vi "DiffDriveSim_Write_Sensors.vi"(6 "Restart":bool, 8 "Right Encoder":T2, 9 "Left Encoder":T2, 10 "Diff Drive Train Sim":T11 {"m_Motor"."Jr_KgM2" format="%13.5p"; "m_Motor"."L_H" format="%13.5p"; "m_Motor"."Kt_NMPerAmp" format="%13.5p"; "m_Motor"."KvINV_RadPerSecPerVolt" format="%13.5p"; "m_Motor"."R_Ohms" format="%13.5p"; "m_Motor"."FreeSpeed_RadPerSec" format="%13.5p"; "m_Motor"."FreeCurrent_Amps" format="%13.5p"; "m_Motor"."StallCurrent_Amps" format="%13.5p"; "m_Motor"."StallTorque_NM" format="%13.5p"; "m_Motor"."nominalVoltage_Volts" format="%13.5p"}, 11 "Counts/Feet":dbl) -> (0 "Right Encoder":T1, 1 "Right Encoder":T9, 2 "Left Encoder":T1, 3 "Left Encoder":T9, 4 "Robot Pose":T6 {"ROTATION"."SIN" format="%13.4f"; "ROTATION"."COS" format="%13.4f"; "ROTATION"."VALUE" format="%13.4f"; "TRANSLATION"."Y" format="%14.3f"; "TRANSLATION"."X" format="%14.3f"}, 5 "Gyro Deg":dbl, 7 "Gyro":T4)   [LabVIEW 2019]
uses:
  <vilib>/Rock Robotics/WPI/ThirdParty/JAS_Junk/TrajLib/TypeDef/DIFF_DRIVE_TRAIN_SIM.ctl
  <vilib>/Rock Robotics/WPI/ThirdParty/JAS_Junk/TrajLib/TypeDef/LINEAR_SYSTEM.ctl
  <vilib>/Analysis/Matrix/Datatypes/RealMatrix.ctl
  <vilib>/Rock Robotics/WPI/ThirdParty/JAS_Junk/TrajLib/TypeDef/DCMOTOR.CTL
  <vilib>/Rock Robotics/WPI/Simulation/Protocol/Devices/Encoder/Encoder proto.ctl
  <vilib>/Rock Robotics/WPI/Simulation/Protocol/Devices/Encoder/Encoder data protoo.ctl
  <vilib>/Rock Robotics/WPI/ThirdParty/JAS_Junk/TrajLib/TypeDef/POSE2D.ctl
  <vilib>/Rock Robotics/WPI/ThirdParty/JAS_Junk/TrajLib/TypeDef/TRANSLATION2D.ctl
  <vilib>/Rock Robotics/WPI/ThirdParty/JAS_Junk/TrajLib/TypeDef/ROTATION2D.ctl
  <vilib>/Rock Robotics/WPI/Simulation/Protocol/Devices/Gyro/Gyro proto.ctl
  <vilib>/Rock Robotics/WPI/Simulation/Protocol/Devices/Gyro/Gyro Data proto.ctl
  DiffDriveSim_EncoderDIOType.ctl
  <vilib>/Rock Robotics/SystemInterfaces/DIO/FPGA_DIOChannel.ctl
  DiffDriveSim_EncoderValues.ctl
  <vilib>/Rock Robotics/WPI/Simulation/Protocol/Devices/Gyro/Gyro Update Ops.ctl
  <vilib>/Rock Robotics/WPI/Simulation/Protocol/Devices/Encoder/Encoder Values.ctl
  <vilib>/Rock Robotics/WPI/Simulation/Protocol/Devices/Encoder/Encoder Update Ops.ctl
  DiffDriveSim_GetAllEncoderInx.vi
  <vilib>/Rock Robotics/SystemInterfaces/FPGA_NIFPGAInterfaceFPGAResourceConstant.vi
  <vilib>/Rock Robotics/SystemInterfaces/Encoder/FPGA_EncoderIdx.ctl
  <vilib>/Rock Robotics/WPI/ThirdParty/JAS_Junk/TrajLib/Trajectory_Library.lvlib
  <vilib>/Analysis/Matrix/NI_Matrix.lvlib
panel:
  out "Right Enc Found":bool
  out "Left Enc Found":bool
  # "<States, 1>"
  # "<Outputs, 1>"
  # "<Inputs, 1>"
  # "<Outputs, 1>"
  # "<States,States>"
  # "<States,Inputs>"
  # "<Outputs,States>"
  # "<Outputs,Inputs>"
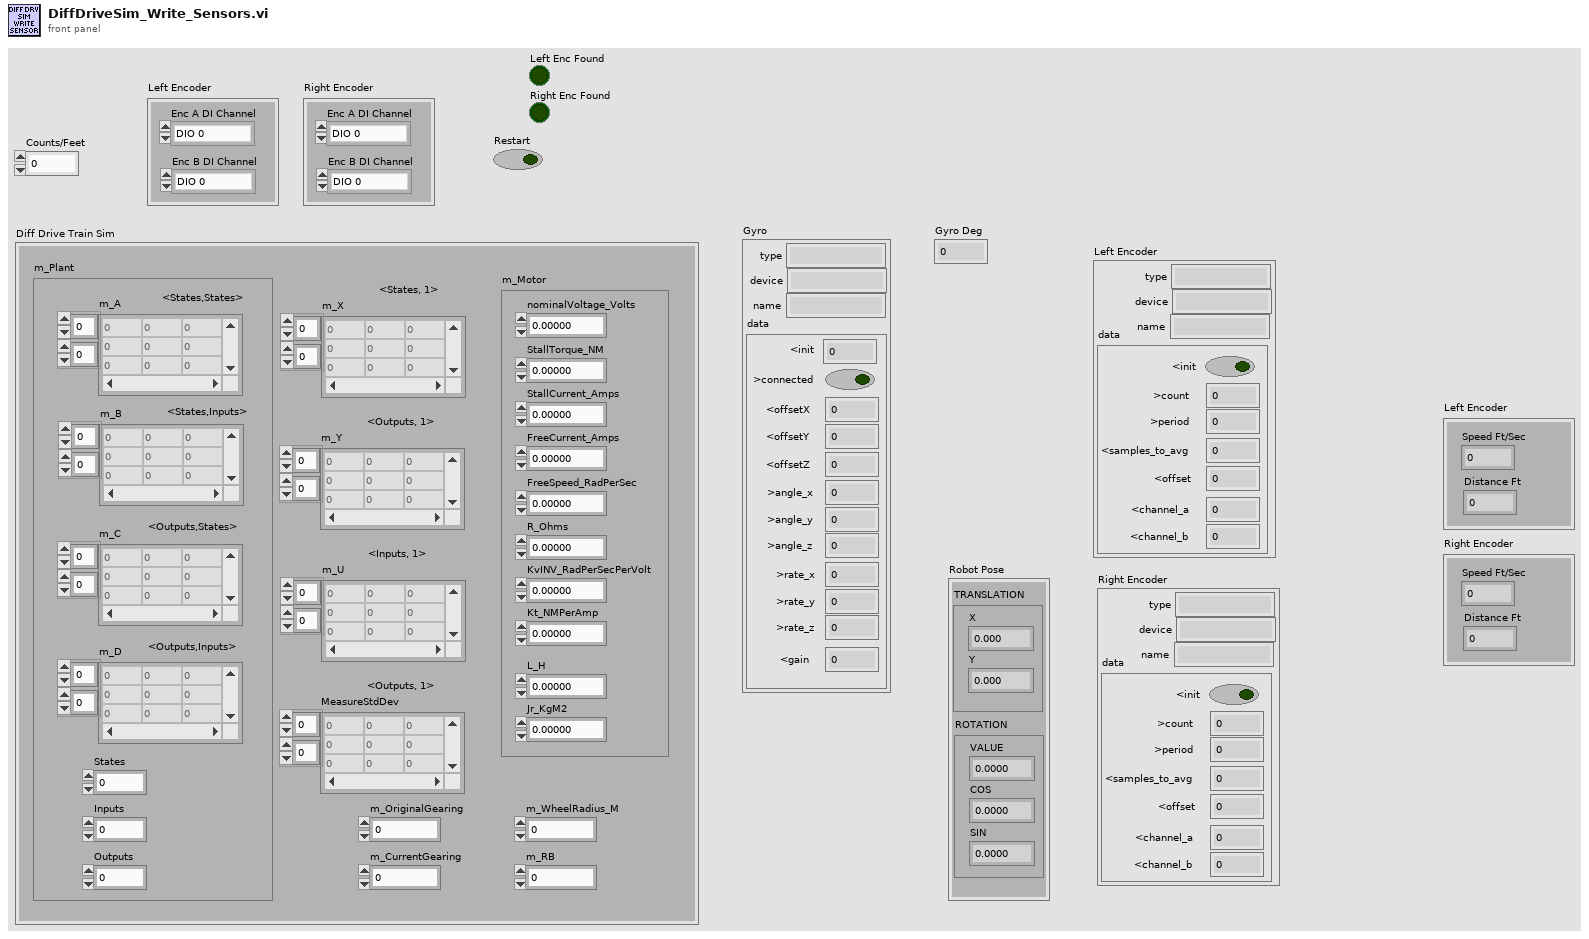
[diagram p1: front panel]
types:
  T1 = typedef "DiffDriveSim_EncoderValues.ctl" = cluster{"Speed Ft/Sec":dbl, "Distance Ft":dbl}
  T2 = typedef "DiffDriveSim_EncoderDIOType.ctl" = cluster{"Enc A DI Channel":T3, "Enc B DI Channel":T3}
  T3 = typedef "FPGA_DIOChannel.ctl" = enum8{"DIO 0", "DIO 1", "DIO 2", "DIO 3", "DIO 4", "DIO 5", "DIO 6", "DIO 7", "DIO 8", "DIO 9", "DIO MXP 0", "DIO MXP 1", "DIO MXP 2", "DIO MXP 3", "DIO MXP 4", "DIO MXP 5", "DIO MXP 6", "DIO MXP 7", "DIO MXP 8", "DIO MXP 9", "DIO MXP 10", "DIO MXP 11", "DIO MXP 12", "DIO MXP 13", "DIO MXP 14", "DIO MXP 15", "SPI Port CS1", "SPI Port CS2", "SPI Port CS3", "SPI Port MISO", "SPI Port MOSI", "Invalid"}
  T4 = typedef "Gyro proto.ctl" = cluster{"type":string, "device":string, "name":string, "data":T5}
  T5 = typedef "Gyro Data proto.ctl" = cluster{"<init":i32, ">connected":bool, "<offsetX":dbl, "<offsetY":dbl, "<offsetZ":dbl, ">angle_x":dbl, ">angle_y":dbl, ">angle_z":dbl, ">rate_x":dbl, ">rate_y":dbl, ">rate_z":dbl, "<gain":dbl}
  T6 = typedef "Trajectory_Library.lvlib/POSE2D.ctl" = cluster{"TRANSLATION":T7, "ROTATION":T8}
  T7 = typedef "Trajectory_Library.lvlib/TRANSLATION2D.ctl" = cluster{"X":dbl, "Y":dbl}
  T8 = typedef "Trajectory_Library.lvlib/ROTATION2D.ctl" = cluster{"VALUE":dbl, "COS":dbl, "SIN":dbl}
  T9 = typedef "Encoder proto.ctl" = cluster{"type":string, "device":string, "name":string, "data":T10}
  T10 = typedef "Encoder data protoo.ctl" = cluster{"<init":bool, ">count":dbl, ">period":dbl, "<samples_to_avg":i32, "<offset":dbl, "<channel_a":i32, "<channel_b":i32}
  T11 = typedef "Trajectory_Library.lvlib/DIFF_DRIVE_TRAIN_SIM.ctl" = cluster{"m_Plant":T12, "m_X":T13, "m_Y":T13, "m_U":T13, "MeasureStdDev":T13, "m_Motor":T14, "m_OriginalGearing":dbl, "m_CurrentGearing":dbl, "m_WheelRadius_M":dbl, "m_RB":dbl}
  T12 = typedef "Trajectory_Library.lvlib/LINEAR_SYSTEM.ctl" = cluster{"m_A":T13, "m_B":T13, "m_C":T13, "m_D":T13, "States":i32, "Inputs":i32, "Outputs":i32}
  T13 = typedef "NI_Matrix.lvlib/RealMatrix.ctl" = dbl[][]
  T14 = typedef "Trajectory_Library.lvlib/DCMOTOR.CTL" = cluster{"nominalVoltage_Volts":dbl, "StallTorque_NM":dbl, "StallCurrent_Amps":dbl, "FreeCurrent_Amps":dbl, "FreeSpeed_RadPerSec":dbl, "R_Ohms":dbl, "KvINV_RadPerSecPerVolt":dbl, "Kt_NMPerAmp":dbl, "L_H":dbl, "Jr_KgM2":dbl}
  T15 = typedef "Gyro Update Ops.ctl" = enum16{"get", "delete", "JSON update", "set  name", "transmit initial", "reset", "set init", "set offsetX", "set offsetY", "set offsetZ", "set gain", "set angle X", "set angle Y", "set angle Z", "set rate X", "set rate Y", "set rate Z"}
  T16 = typedef "Encoder Update Ops.ctl" = enum16{"set init", "set count", "set period", "set reset", "set samples_to_avg", "get", "delete", "JSON update", "set name", "transmit initial", "reset", "set channel_a", "set channel_b", "set values"}
  T17 = typedef "FPGA_EncoderIdx.ctl" = enum8{"Enc 0", "Enc 1", "Enc 2", "Enc 3", "Enc 4", "Enc 5", "Enc 6", "Enc 7", "Invalid"}
  T18 = typedef "Encoder Values.ctl" = cluster{"Count":dbl, "Period":dbl}
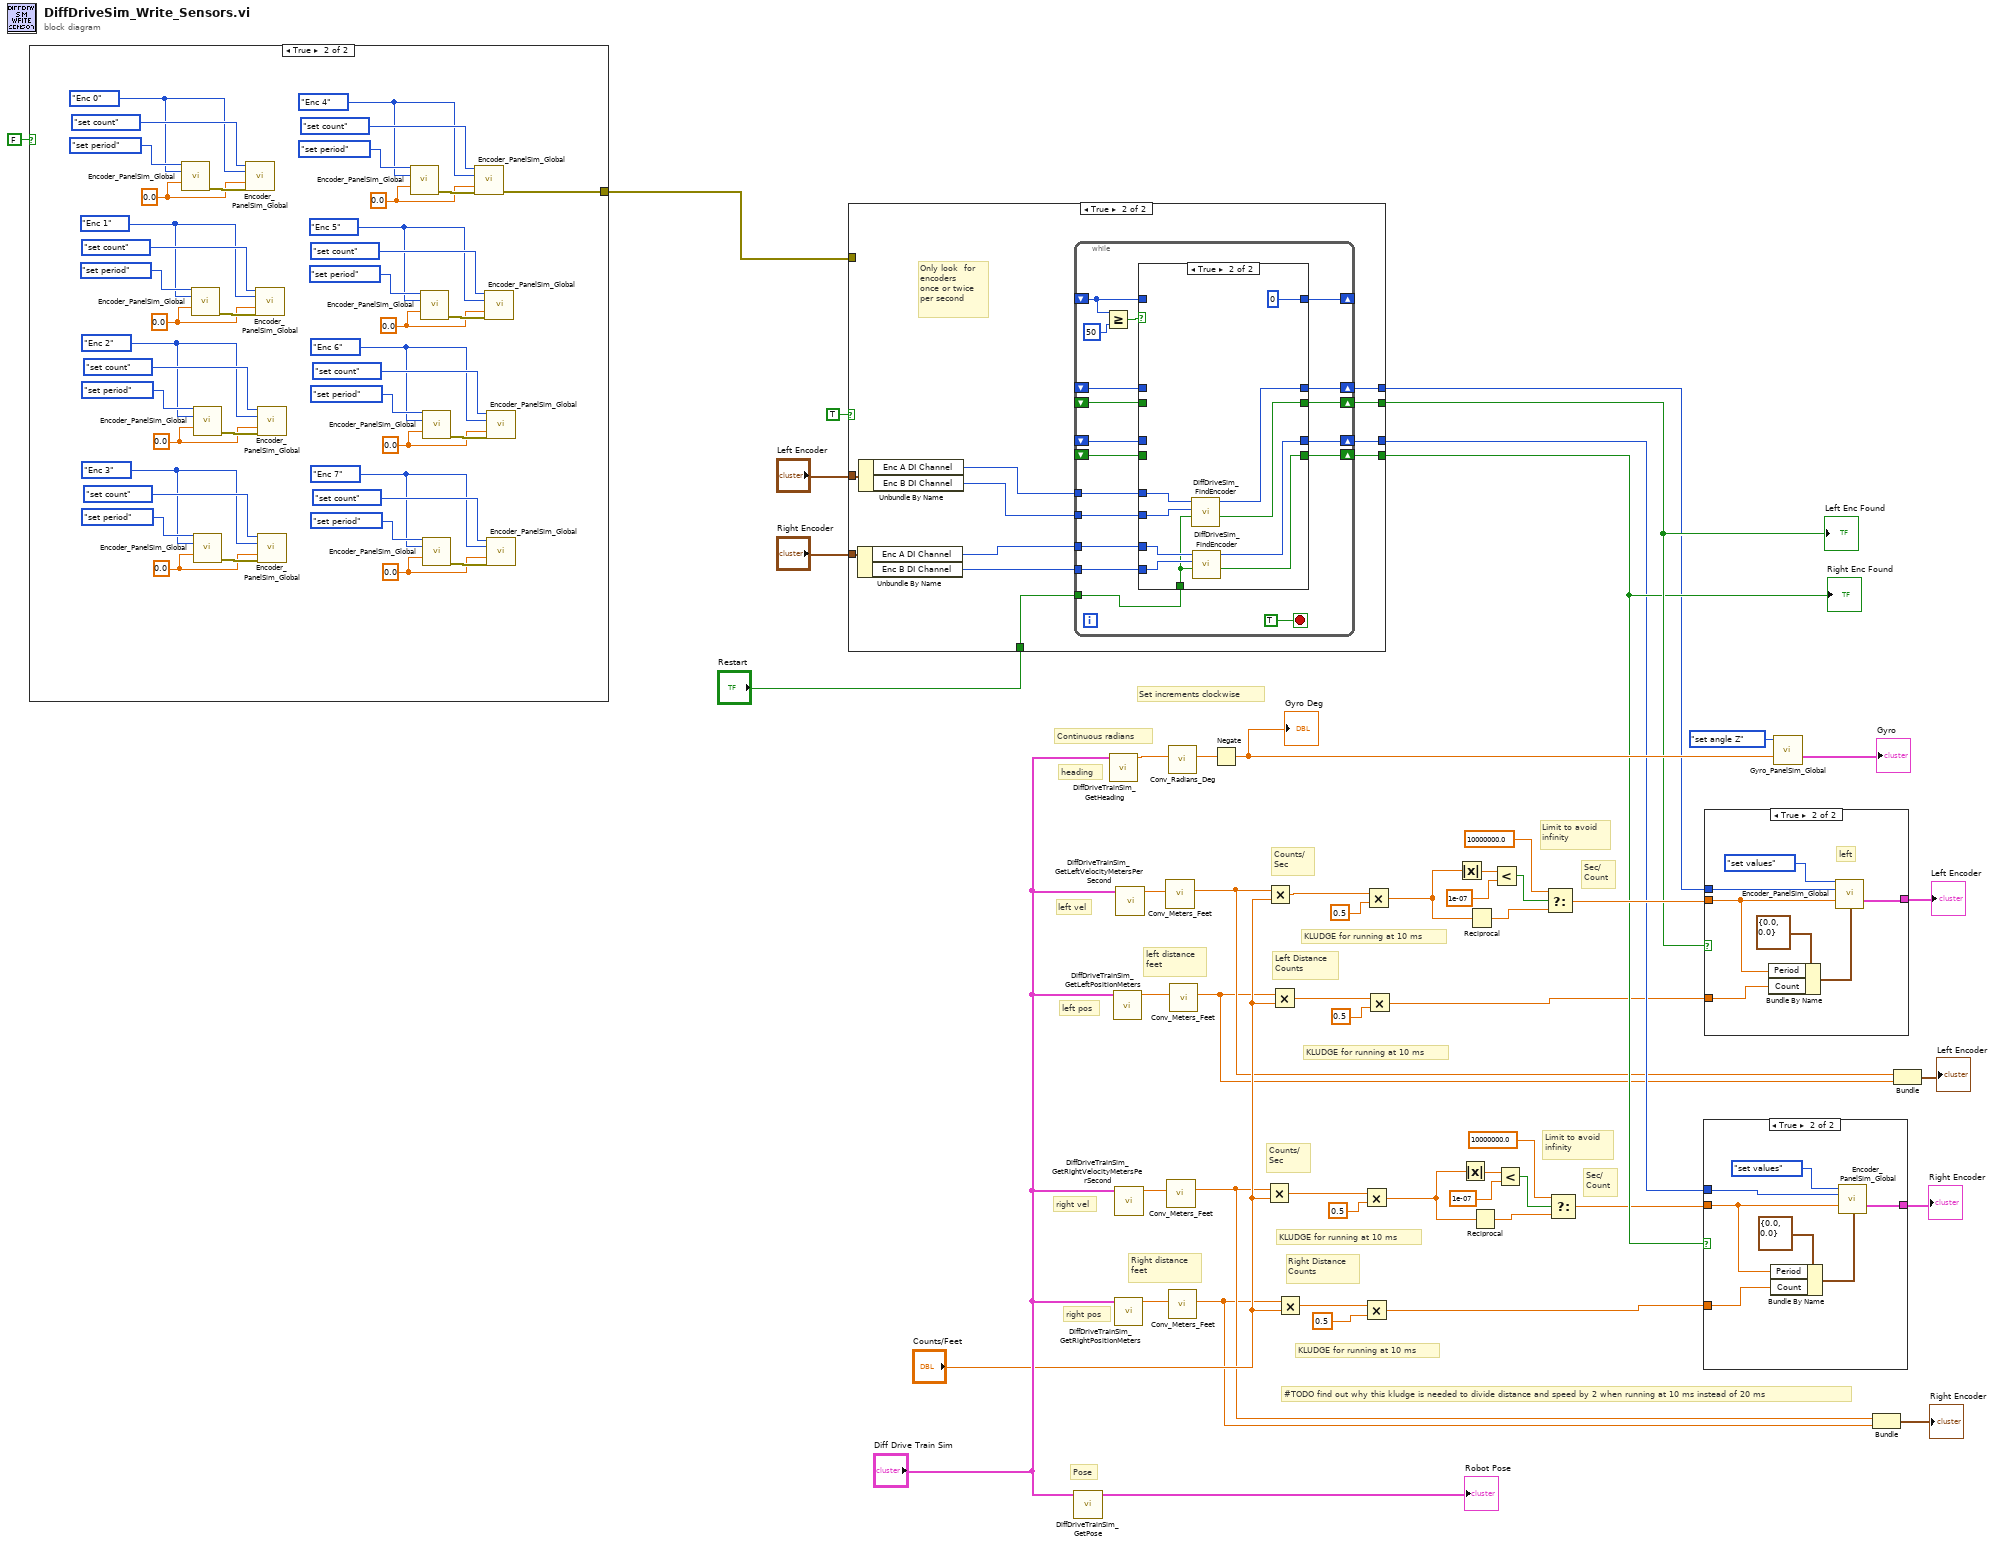
[diagram p0: block diagram]
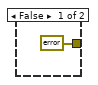
[diagram p2: hidden frame]
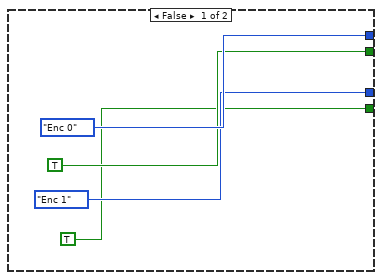
[diagram p3: hidden frame]
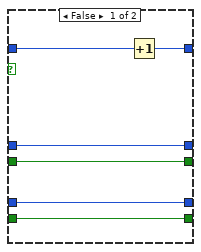
[diagram p4: hidden frame]
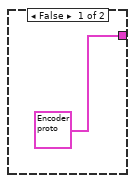
[diagram p5: hidden frame]
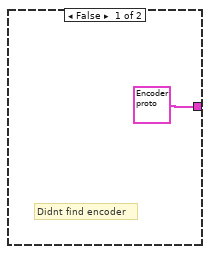
[diagram p6: hidden frame]
diagram:
  # "KLUDGE for running at 10 ms"
  # "KLUDGE for running at 10 ms"
  # "Counts/\nSec"
  # "Limit to avoid\ninfinity"
  # "Sec/\nCount"
  # "KLUDGE for running at 10 ms"
  # "KLUDGE for running at 10 ms"
  # "#TODO find out why this kludge is needed to divide distance and speed by 2 when running at 10 ms instead of 20 ms"
  # "Set increments clockwise"
  # "Limit to avoid\ninfinity"
  # "Right Distance\nCounts"
  # "Left Distance\nCounts"
  # "Sec/\nCount"
  # "Counts/\nSec"
  # "Continuous radians"
  # "Right distance\nfeet"
  # "left distance\nfeet"
  # "heading"
  # "left pos"
  # "right pos"
  # "right vel"
  # "left vel"
  # "Pose"
  n1 = case shown="True" FALSE {
    tunnel: [errorcluster {"status"=FALSE, "code"=0, "source"=""} ("error out") w56] -> w30
    frame False {
    }
    frame True {
      w58 = 0.0 ("Numeric Value")
      w57 = FPGA_EncoderIdx."Enc 7" ("EncoderIndex")
      w63 = 0.0 ("Numeric Value")
      w62 = FPGA_EncoderIdx."Enc 6" ("EncoderIndex")
      w68 = 0.0 ("Numeric Value")
      w67 = FPGA_EncoderIdx."Enc 5" ("EncoderIndex")
      w73 = 0.0 ("Numeric Value")
      w72 = FPGA_EncoderIdx."Enc 4" ("EncoderIndex")
      w78 = 0.0 ("Numeric Value")
      w77 = FPGA_EncoderIdx."Enc 3" ("EncoderIndex")
      w83 = 0.0 ("Numeric Value")
      w82 = FPGA_EncoderIdx."Enc 2" ("EncoderIndex")
      w88 = 0.0 ("Numeric Value")
      w87 = FPGA_EncoderIdx."Enc 1" ("EncoderIndex")
      w93 = 0.0 ("Numeric Value")
      w92 = FPGA_EncoderIdx."Enc 0" ("EncoderIndex")
      n2 = call <vilib>:"Encoder_PanelSim_Global.vi"("menu"=Encoder_Update_Ops."set period", "EncoderIndex"=w92, "Numeric Value"=w93) -> ("error out"=w96:errorcluster)  [unwired: 11 in, 1 out]
      n3 = call <vilib>:"Encoder_PanelSim_Global.vi"("menu"=Encoder_Update_Ops."set period", "EncoderIndex"=w87, "Numeric Value"=w88) -> ("error out"=w91:errorcluster)  [unwired: 11 in, 1 out]
      n4 = call <vilib>:"Encoder_PanelSim_Global.vi"("menu"=Encoder_Update_Ops."set period", "EncoderIndex"=w82, "Numeric Value"=w83) -> ("error out"=w86:errorcluster)  [unwired: 11 in, 1 out]
      n5 = call <vilib>:"Encoder_PanelSim_Global.vi"("menu"=Encoder_Update_Ops."set period", "EncoderIndex"=w77, "Numeric Value"=w78) -> ("error out"=w81:errorcluster)  [unwired: 11 in, 1 out]
      n6 = call <vilib>:"Encoder_PanelSim_Global.vi"("menu"=Encoder_Update_Ops."set count", "EncoderIndex"=w92, "Numeric Value"=w93, "error in (no error)"=w96) -> ()  [unwired: 10 in, 2 out]
      n7 = call <vilib>:"Encoder_PanelSim_Global.vi"("menu"=Encoder_Update_Ops."set count", "EncoderIndex"=w87, "Numeric Value"=w88, "error in (no error)"=w91) -> ()  [unwired: 10 in, 2 out]
      n8 = call <vilib>:"Encoder_PanelSim_Global.vi"("menu"=Encoder_Update_Ops."set count", "EncoderIndex"=w82, "Numeric Value"=w83, "error in (no error)"=w86) -> ()  [unwired: 10 in, 2 out]
      n9 = call <vilib>:"Encoder_PanelSim_Global.vi"("menu"=Encoder_Update_Ops."set count", "EncoderIndex"=w77, "Numeric Value"=w78, "error in (no error)"=w81) -> ()  [unwired: 10 in, 2 out]
      n10 = call <vilib>:"Encoder_PanelSim_Global.vi"("menu"=Encoder_Update_Ops."set period", "EncoderIndex"=w72, "Numeric Value"=w73) -> ("error out"=w76:errorcluster)  [unwired: 11 in, 1 out]
      n11 = call <vilib>:"Encoder_PanelSim_Global.vi"("menu"=Encoder_Update_Ops."set period", "EncoderIndex"=w67, "Numeric Value"=w68) -> ("error out"=w71:errorcluster)  [unwired: 11 in, 1 out]
      n12 = call <vilib>:"Encoder_PanelSim_Global.vi"("menu"=Encoder_Update_Ops."set period", "EncoderIndex"=w62, "Numeric Value"=w63) -> ("error out"=w66:errorcluster)  [unwired: 11 in, 1 out]
      n13 = call <vilib>:"Encoder_PanelSim_Global.vi"("menu"=Encoder_Update_Ops."set period", "EncoderIndex"=w57, "Numeric Value"=w58) -> ("error out"=w61:errorcluster)  [unwired: 11 in, 1 out]
      n14 = call <vilib>:"Encoder_PanelSim_Global.vi"("menu"=Encoder_Update_Ops."set count", "EncoderIndex"=w72, "Numeric Value"=w73, "error in (no error)"=w76) -> ("error out"=w56:errorcluster)  [unwired: 10 in, 1 out]
      n15 = call <vilib>:"Encoder_PanelSim_Global.vi"("menu"=Encoder_Update_Ops."set count", "EncoderIndex"=w67, "Numeric Value"=w68, "error in (no error)"=w71) -> ()  [unwired: 10 in, 2 out]
      n16 = call <vilib>:"Encoder_PanelSim_Global.vi"("menu"=Encoder_Update_Ops."set count", "EncoderIndex"=w62, "Numeric Value"=w63, "error in (no error)"=w66) -> ()  [unwired: 10 in, 2 out]
      n17 = call <vilib>:"Encoder_PanelSim_Global.vi"("menu"=Encoder_Update_Ops."set count", "EncoderIndex"=w57, "Numeric Value"=w58, "error in (no error)"=w61) -> ()  [unwired: 10 in, 2 out]
    }
  }
  n18 = case shown="True" TRUE {
    tunnel: "Right Encoder" -> [_ w111]
    tunnel: "Left Encoder" -> [_ w110]
    tunnel: "Restart" -> [_ w105]
    tunnel: [TRUE ("Found") w104] -> w35
    tunnel: [TRUE ("Found") w103] -> w34
    tunnel: [FPGA_EncoderIdx."Enc 0" ("EncoderIndex") w102] -> w33
    tunnel: [FPGA_EncoderIdx."Enc 1" ("EncoderIndex") w101] -> w32
    tunnel: w30 -> [_ _]
    frame False {
    }
    frame True {
      # "Only look  for\nencoders \nonce or twice\nper second"
      n19 = Unbundle By Name(w111) -> ("Enc A DI Channel"=w107:T3, "Enc B DI Channel"=w106:T3)
      n20 = Unbundle By Name(w110) -> ("Enc A DI Channel"=w109:T3, "Enc B DI Channel"=w108:T3)
      n21 = while {
        tunnel: w109 -> [w129]
        tunnel: w108 -> [w128]
        tunnel: w107 -> [w127]
        tunnel: w106 -> [w126]
        tunnel: w105 -> [w125]
        shift-right: [w117] -> _
        shift-left: _ -> [w112]
        shift-right: [w122] -> w102
        shift-left: _ -> [w116]
        shift-right: [w124] -> w104
        shift-left: _ -> [w115]
        shift-right: [w121] -> w101
        shift-left: _ -> [w114]
        shift-right: [w123] -> w103
        shift-left: _ -> [w113]
        stop <- TRUE stop-if-true
        n22 = Greater Or Equal?(x=w112, y=50) -> (x >= y?=w119:bool)
        n23 = case shown="True" w119 {
          tunnel: w129 -> [_ w145]
          tunnel: w128 -> [_ w144]
          tunnel: w127 -> [_ w143]
          tunnel: w126 -> [_ w142]
          tunnel: w125 -> [_ w141]
          tunnel: [w134 w140] -> w124
          tunnel: [w132 w139] -> w123
          tunnel: [w135 w138] -> w122
          tunnel: [w133 w137] -> w121
          tunnel: [w130 0] -> w117
          tunnel: w116 -> [w135 _]
          tunnel: w115 -> [w134 _]
          tunnel: w114 -> [w133 _]
          tunnel: w113 -> [w132 _]
          tunnel: w112 -> [w131 _]
          frame False {
            n24 = Increment(x=w131) -> (x+1=w130:i32)
          }
          frame True {
            n25 = call "DiffDriveSim_FindEncoder.vi"("Restart"=w141, "Enc B DI Channel"=w144, "Enc A DI Channel"=w145) -> ("Found"=w140:bool, "EncoderIndex"=w138:T17)  [unwired: 7 in]
            n26 = call "DiffDriveSim_FindEncoder.vi"("Restart"=w141, "Enc B DI Channel"=w142, "Enc A DI Channel"=w143) -> ("Found"=w139:bool, "EncoderIndex"=w137:T17)  [unwired: 7 in]
          }
        }
      }
    }
  }
  "Left Enc Found" <- w35
  "Right Enc Found" <- w34
  n27 = call <vilib>:"DiffDriveTrainSim_GetPose.vi"("DiffDriveTrainSim"="Diff Drive Train Sim") -> ("Pose"=→"Robot Pose":T6)  [unwired: 10 in]
  n28 = call <vilib>:"DiffDriveTrainSim_GetHeading.vi"("DiffDriveTrainSim"="Diff Drive Train Sim") -> ("Heading"=w52:dbl)  [unwired: 10 in]
  n29 = call <vilib>:"DiffDriveTrainSim_GetLeftPositionMeters.vi"("DiffDriveTrainSim"="Diff Drive Train Sim") -> ("LeftPosition_Meters"=w48:dbl)  [unwired: 10 in]
  n30 = call <vilib>:"DiffDriveTrainSim_GetRightPositionMeters.vi"("DiffDriveTrainSim"="Diff Drive Train Sim") -> ("RightPosition_Meters"=w45:dbl)  [unwired: 10 in]
  n31 = call <vilib>:"DiffDriveTrainSim_GetRightVelocityMetersPerSecond.vi"("DiffDriveTrainSim"="Diff Drive Train Sim") -> ("RightVel_M_Per_Sec"=w46:dbl)  [unwired: 10 in]
  n32 = call <vilib>:"DiffDriveTrainSim_GetLeftVelocityMetersPerSecond.vi"("DiffDriveTrainSim"="Diff Drive Train Sim") -> ("LeftVelocity_M_Per_Sec"=w47:dbl)  [unwired: 10 in]
  n33 = call <vilib>:"Conv_Meters_Feet.vi"("Meters"=w47) -> ("Feet"=w27:dbl)  [unwired: 10 in]
  n34 = call <vilib>:"Conv_Meters_Feet.vi"("Meters"=w46) -> ("Feet"=w25:dbl)  [unwired: 10 in]
  n35 = call <vilib>:"Conv_Radians_Deg.vi"("Radians"=w52) -> ("Degrees"=w40:dbl)  [unwired: 10 in]
  n36 = call <vilib>:"Conv_Meters_Feet.vi"("Meters"=w45) -> ("Feet"=w24:dbl)  [unwired: 10 in]
  n37 = call <vilib>:"Conv_Meters_Feet.vi"("Meters"=w48) -> ("Feet"=w26:dbl)  [unwired: 10 in]
  n38 = Negate(x=w40) -> (-x=w39:dbl)
  "Gyro Deg" <- w39
  n39 = Multiply(x=w25, y="Counts/Feet") -> (x*y=w2:dbl)
  n40 = Multiply(x=w27, y="Counts/Feet") -> (x*y=w5:dbl)
  n41 = Multiply(x=w26, y="Counts/Feet") -> (x*y=w20:dbl)
  n42 = Multiply(x=w24, y="Counts/Feet") -> (x*y=w17:dbl)
  n43 = Multiply(x=w2, y=0.5) -> (x*y=w1:dbl)
  n44 = Multiply(x=w17, y=0.5) -> (x*y=w18:dbl)
  n45 = Multiply(x=w5, y=0.5) -> (x*y=w4:dbl)
  n46 = Multiply(x=w20, y=0.5) -> (x*y=w22:dbl)
  n47 = Absolute Value(x=w4) -> (abs(x)=w16:dbl)
  n48 = Absolute Value(x=w1) -> (abs(x)=w11:dbl)
  n49 = Reciprocal(x=w4) -> (1/x=w14:dbl)
  n50 = Reciprocal(x=w1) -> (1/x=w9:dbl)
  n51 = Less?(x=w16, y=1e-07) -> (x < y?=w13:bool)
  n52 = Less?(x=w11, y=1e-07) -> (x < y?=w8:bool)
  n53 = Select(t=10000000.0, s=w13, f=w14) -> (s? t:f=w43:dbl)
  n54 = Select(t=10000000.0, s=w8, f=w9) -> (s? t:f=w7:dbl)
  n55 = case shown="True" w34 {
    tunnel: [T9 {"type"="Encoder", "device"="", "name"="", "data"={"<init"=FALSE, ">count"=0.0, ">period"=0.0, "<samples_to_avg"=0, "<offset"=0.0, "<channel_a"=0, "<channel_b"=0}} ("Encoder new") w151] -> w51
    tunnel: w18 -> [_ w148]
    tunnel: w7 -> [_ w149]
    tunnel: w32 -> [_ w152]
    frame False {
    }
    frame True {
      n56 = Bundle By Name(cluster=T18 {"Count"=0.0, "Period"=0.0} ("Encoder Values"), "Period"=w149, "Count"=w148) -> (w147:T18)
      n57 = call <vilib>:"Encoder_PanelSim_Global.vi"("menu"=Encoder_Update_Ops."set values", "EncoderIndex"=w152, "Numeric Value"=w149, "Values"=w147) -> ("Encoder new"=w151:T9)  [unwired: 10 in, 1 out]
    }
  }
  "Right Encoder" <- w51
  n58 = case shown="True" w35 {
    tunnel: [T9 {"type"="Encoder", "device"="", "name"="", "data"={"<init"=FALSE, ">count"=0.0, ">period"=0.0, "<samples_to_avg"=0, "<offset"=0.0, "<channel_a"=0, "<channel_b"=0}} ("Encoder new") w159] -> w50
    tunnel: w22 -> [_ w156]
    tunnel: w43 -> [_ w157]
    tunnel: w33 -> [_ w160]
    frame False {
      # "Didnt find encoder"
    }
    frame True {
      # "left"
      n59 = Bundle By Name(cluster=T18 {"Count"=0.0, "Period"=0.0} ("Encoder Values"), "Period"=w157, "Count"=w156) -> (w155:T18)
      n60 = call <vilib>:"Encoder_PanelSim_Global.vi"("menu"=Encoder_Update_Ops."set values", "EncoderIndex"=w160, "Numeric Value"=w157, "Values"=w155) -> ("Encoder new"=w159:T9)  [unwired: 10 in, 1 out]
    }
  }
  "Left Encoder" <- w50
  n61 = call <vilib>:"Gyro_PanelSim_Global.vi"("Menu"=Gyro_Update_Ops."set angle Z", "Numeric Value"=w39) -> ("Value out"=→"Gyro":T4)  [unwired: 12 in, 1 out]
  n62 = Bundle("Feet"=w25, "Feet"=w24) -> (→"Right Encoder":cluster{"Feet":dbl, "Feet":dbl})  [unwired: 1 in]
  n63 = Bundle("Feet"=w27, "Feet"=w26) -> (→"Left Encoder":cluster{"Feet":dbl, "Feet":dbl})  [unwired: 1 in]
